vi "SaveConfigCluster.vi"(3 "error in (no error)":errorcluster, 5 "Action":enum16{"Read", "Write"}(ring)) -> (0 "error out":errorcluster, 1 "error?":bool, 2 "message":string=" INSTRUCTIONS:\r\rNormal Use:  When using subVIs that incorporate the error in/error out (or error I/O) structure, place this handler where you want to inform the user of an error, typically at the end of the I/O data path, as the last action of the program.  If the error in error? is ERROR, the handler creates a message describing the error and its source.  If the type of dialog = 1 (default), the message is displayed to the user, who can only acknowedge it.  If the type = 2, the user can acknowledge the message or abort execution; aborting a program with active I/O is not recommended.  If the type = 0, no message is displayed; this is used to process the error programmatically, and the error out cluster elements are wired to individual terminals for that reason.  \r\rOther Use:\n\r\nlocal testing.  To test the error code of a subVI or function that does not have the error I/O structure, you can wire its error code and a source string to the local error code and error source inputs.  If error in error? indicates no error and error code is not equal to 0, the local code and source are substituted for the error in values, and error? is set TRUE (ERROR).")   [LabVIEW 2012]
uses:
  <vilib>/Utility/config.llb/NI_LVConfig.lvlib
  <vilib>/Utility/config.llb/Write Key (I32).vi
  <vilib>/Utility/config.llb/Write Key (Double).vi
  <vilib>/Utility/config.llb/Read Key (I32).vi
  <vilib>/Utility/error.llb/DialogType.ctl
  Config.ctl
panel:
  in  "ConfigRef":refnum<vi>
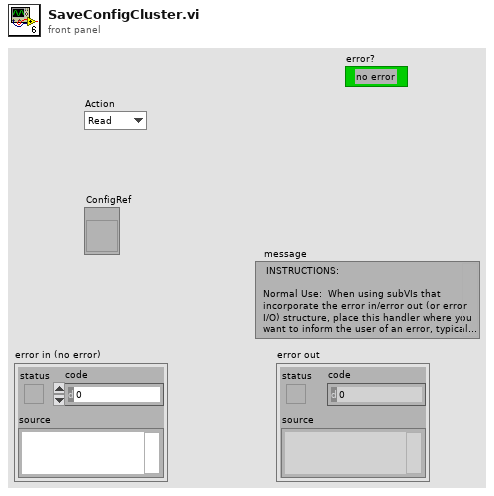
[diagram p1: front panel]
types:
  T1 = typedef "DialogType.ctl" = u16
  T2 = typedef "NI_LVConfig.lvlib/Config Data RefNum.ctl" = refnum<k1>
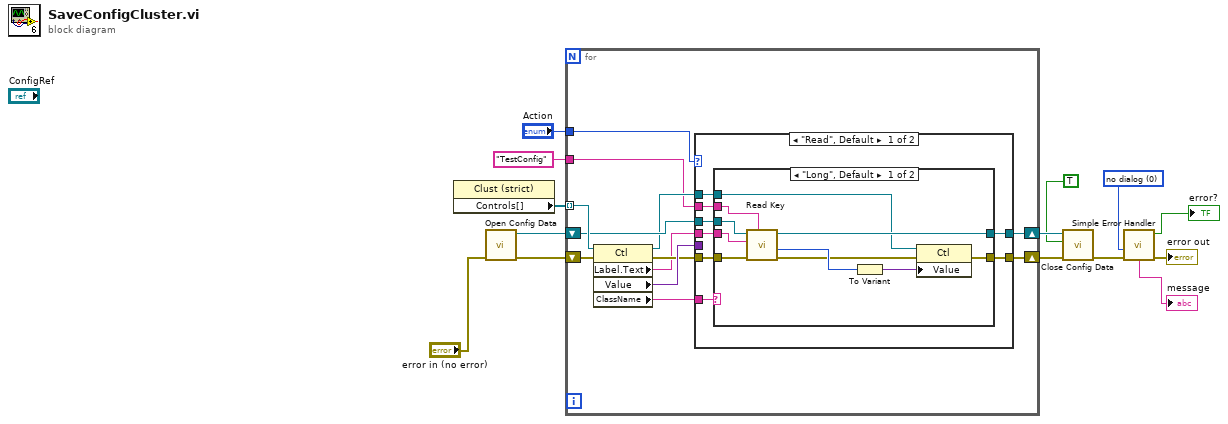
[diagram p0: block diagram]
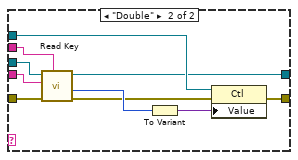
[diagram p2: hidden frame]
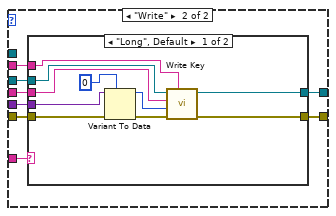
[diagram p3: hidden frame]
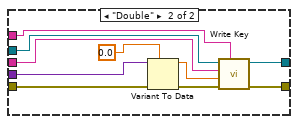
[diagram p4: hidden frame]
diagram:
  w3 = T1 0 items=["no dialog", "OK message", "continue or stop message", "OK message + warnings", "continue/stop + warnings"] ("type of dialog (OK msg:1)")
  n1 = property class="Clust (strict)"() -> (reference=w1:refnum<vi>, "Controls[]"=w2:refnum<vi>[])  [unwired: 1 in, 2 out]
  n2 = call <vilib>:"Open Config Data.vi"("error in (no error)"="error in (no error)") -> ("error out"=w14:errorcluster, "refnum"=w15:T2)  [unwired: 8 in, 1 out]
  n3 = for {
    tunnel: w2 -> [w27] mode=indexing
    shift-right: [w22] -> w11
    shift-left: w14 -> [w23]
    shift-right: [w21] -> w13
    shift-left: w15 -> [w24]
    tunnel: "Action" -> [w20]
    tunnel: "TestConfig" ("section") -> [w18]
    n4 = property class="Ctl"(reference=w27, error in=w23) -> (reference out=w19:refnum<vi>, error out=w25:errorcluster, "Label.Text"=w16:string, "Value"=w26:variant, "ClassName"=w17:string)
    n5 = case shown="\"Read\", Default" w20 {
      tunnel: w26 -> [_ w63]
      tunnel: w25 -> [w34 w62]
      tunnel: w24 -> [w35 w61]
      tunnel: [w32 w60] -> w22
      tunnel: [w31 w59] -> w21
      tunnel: w19 -> [w33 _]
      tunnel: w18 -> [w29 w58]
      tunnel: w17 -> [w30 w57]
      tunnel: w16 -> [w28 w56]
      frame "Read", Default {
        n6 = case shown="\"Long\", Default" w30 {
          tunnel: [w38 w48] -> w32
          tunnel: [w43 w49] -> w31
          tunnel: w35 -> [w45 w52]
          tunnel: w34 -> [w44 w50]
          tunnel: w33 -> [w40 w51]
          tunnel: w29 -> [w37 w47]
          tunnel: w28 -> [w36 w46]
          frame "Long", Default {
            n7 = call-poly <vilib>:"Read Key.vi"("section"=w37, "error in (no error)"=w44, "key"=w36, "refnum"=w45) -> ("error out"=w39:errorcluster, "value"=w41:i32, "refnum out"=w43:T2)  [unwired: 1 in, 4 out]
            n8 = To Variant(anything=w41) -> (Variant=w42:variant)
            n9 = property class="Ctl"(reference=w40, error in=w39, "Value"=w42) -> (error out=w38:errorcluster)  [unwired: 1 out]
          }
          frame "Double" {
            n10 = call-poly <vilib>:"Read Key.vi"("section"=w47, "error in (no error)"=w50, "key"=w46, "refnum"=w52) -> ("error out"=w53:errorcluster, "value"=w54:i32, "refnum out"=w49:T2)  [unwired: 1 in, 4 out]
            n11 = To Variant(anything=w54) -> (Variant=w55:variant)
            n12 = property class="Ctl"(reference=w51, error in=w53, "Value"=w55) -> (error out=w48:errorcluster)  [unwired: 1 out]
          }
        }
      }
      frame "Write" {
        n13 = case shown="\"Long\", Default" w57 {
          tunnel: w63 -> [w73 w82]
          tunnel: w62 -> [w71 w81]
          tunnel: [w68 w77] -> w60
          tunnel: w61 -> [w67 w78]
          tunnel: [w66 w76] -> w59
          tunnel: w58 -> [w65 w75]
          tunnel: w56 -> [w64 w74]
          frame "Long", Default {
            n14 = Variant To Data(error in=w71, type=0, Variant=w73) -> (data=w70:i32, error out=w69:errorcluster)
            n15 = call-poly <vilib>:"Write Key.vi"("section"=w65, "error in (no error)"=w69, "value"=w70, "key"=w64, "refnum"=w67) -> ("error out"=w68:errorcluster, "refnum out"=w66:T2)  [unwired: 4 in, 1 out]
          }
          frame "Double" {
            n16 = Variant To Data(error in=w81, type=0.0, Variant=w82) -> (data=w80:dbl, error out=w79:errorcluster)
            n17 = call-poly <vilib>:"Write Key.vi"("section"=w75, "error in (no error)"=w79, "value"=w80, "key"=w74, "refnum"=w78) -> ("error out"=w77:errorcluster, "refnum out"=w76:T2)  [unwired: 4 in, 1 out]
          }
        }
      }
    }
  }
  n18 = call <vilib>:"Close Config Data.vi"("error in (no error)"=w11, "write file if changed (T)"=TRUE, "refnum"=w13) -> ("error out"=w7:errorcluster)  [unwired: 8 out]
  n19 = call <vilib>:"Simple Error Handler.vi"("type of dialog (OK msg:1)"=w3, "error in (no error)"=w7) -> ("error?"=→"error?":bool, "error out"=→"error out":errorcluster, "message"=→"message":string)  [unwired: 3 in, 2 out]
